vi "close_hw.vi"(8 "error in (no error)":errorcluster, 11 "XPS control in":refnum<class "XPS.lvclass">) -> (0 "error out":errorcluster, 3 "XPS control out":refnum<class "XPS.lvclass">)   [LabVIEW 2019, in "XPS.lvlib" / "XPS.lvclass"]
uses:
  XPS.lvclass
  XPS.lvclass/XPS.ctl
  Newport.XPS.CommandInterface
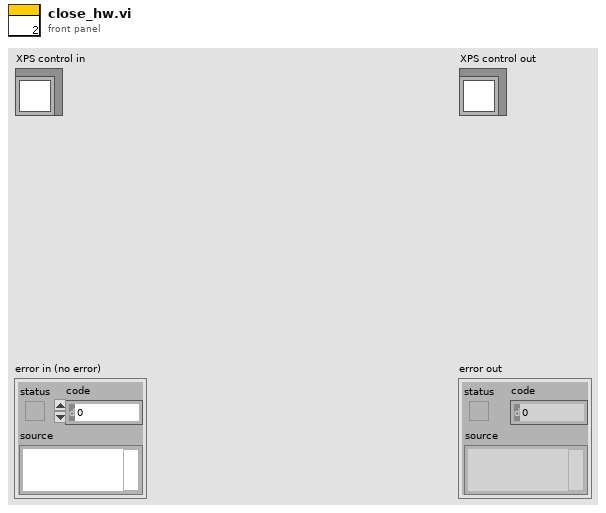
[diagram p1: front panel]
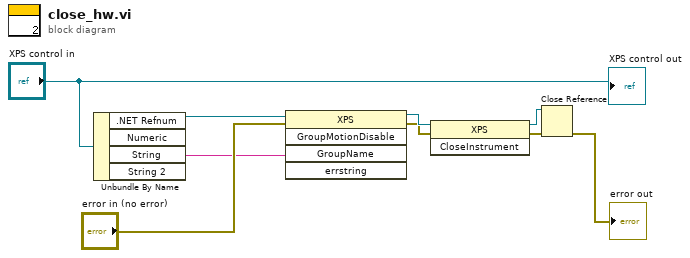
[diagram p0: block diagram]
diagram:
  n1 = Unbundle By Name("XPS control in") -> (".NET Refnum"=w4:refnum<k24>, "String"=w1:string)  [unwired: 2 out]
  n2 = invoke class="XPS" method="GroupMotionDisable"(reference=w4, error in="error in (no error)", "GroupName"=w1) -> (reference out=w7:refnum<k24>, error out=w6:errorcluster)  [unwired: 2 in, 3 out]
  n3 = invoke class="XPS" method="CloseInstrument"(reference=w7, error in=w6) -> (reference out=w8:refnum<k24>, error out=w9:errorcluster)  [unwired: 1 in, 1 out]
  n4 = Close Reference(reference=w8, error in (no error)=w9) -> (error out=→"error out":errorcluster)
  "XPS control out" <- "XPS control in"
